vi "GCMBuilder.vi"() -> ()   [LabVIEW 2014]
uses:
  <vilib>/JKI/VIPM API/command-line/support/Version Info Cluster_vipm_api.ctl
  <vilib>/JKI/VIPM API/VIPM API_vipm_api.lvlib
panel:
  out "Build Output":path
  in  "Build":bool
  in  "VI Package Build Spec Data":T2
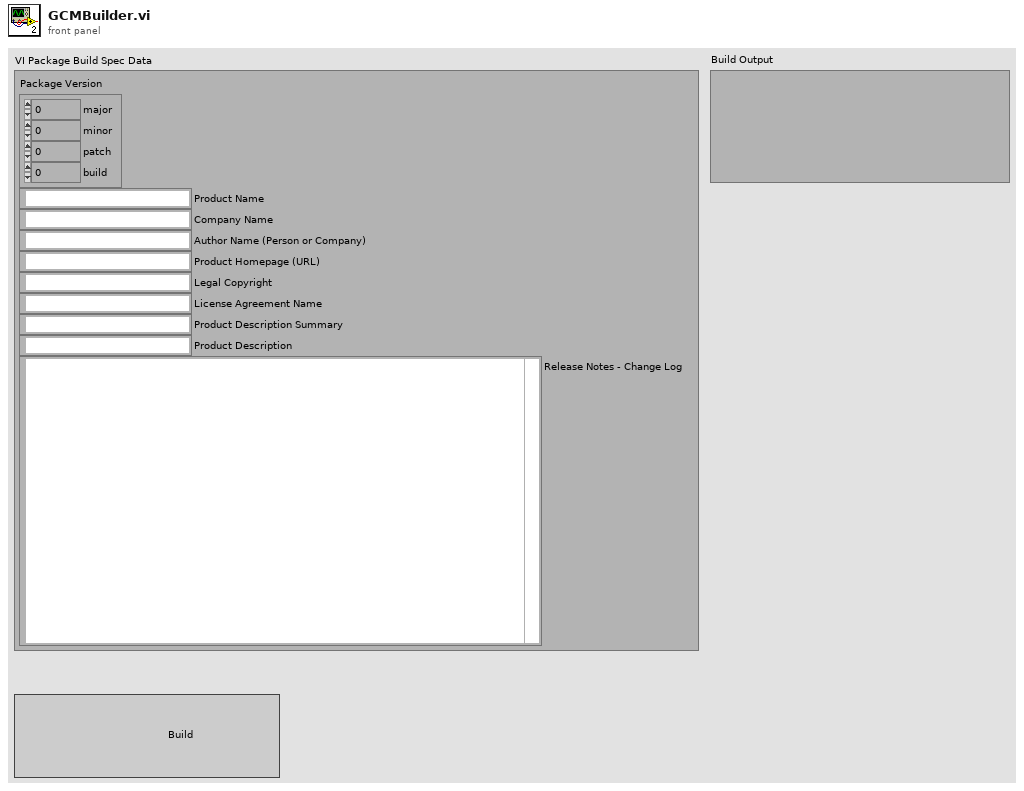
[diagram p1: front panel]
types:
  T1 = typedef "VIPM API_vipm_api.lvlib/Version Info Cluster_vipm_api.ctl" = cluster{"major":u32, "minor":u32, "patch":u32, "build":u32}
  T2 = cluster{"Package Version":T1, "Product Name":string, "Company Name":string, "Author Name (Person or Company)":string, "Product Homepage (URL)":string, "Legal Copyright":string, "License Agreement Name":string, "Product Description Summary":string, "Product Description":string, "Release Notes - Change Log":string}
  T3 = typedef "VIPM API_vipm_api.lvlib/VI Package Build Spec Data Cluster_vipm_api.ctl" = cluster{"Package Version":T1, "Product Name":string, "Company Name":string, "Author Name (Person or Company)":string, "Product Homepage (URL)":string, "Legal Copyright":string, "License Agreement Name":string, "Product Description Summary":string, "Product Description":string, "Release Notes - Change Log":string}
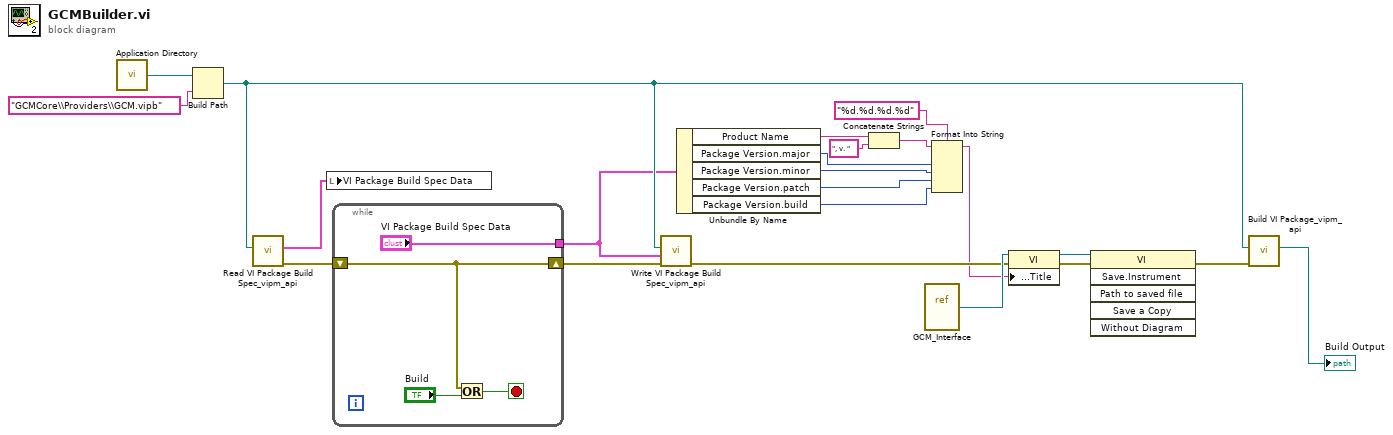
[diagram p0: block diagram]
diagram:
  n1 = call <vilib>:"Application Directory.vi"() -> ("Application Directory"=w22:path)
  n2 = Build Path(base path=w22, name or relative path="GCMCore\\Providers\\GCM.vipb") -> (appended path=w3:path)
  n3 = call <vilib>:"Read VI Package Build Spec_vipm_api.vi"("Path to VIPB File"=w3) -> ("error out"=w20:errorcluster, "VI Package Build Spec Data"=w4:T3)  [unwired: 9 in]
  n4 = local write "VI Package Build Spec Data"(w4) -> ()
  n5 = while {
    shift-right: [w26] -> w19
    shift-left: w20 -> [w26]
    tunnel: ["VI Package Build Spec Data"] -> w1
    stop <- w24 stop-if-true
    n6 = Or(x=w26, y="Build") -> (x .or. y?=w24:bool)
  }
  n7 = call <vilib>:"Write VI Package Build Spec_vipm_api.vi"("error in (no error)"=w19, "VI Package Build Spec Data"=w1, "Path to VIPB File"=w3) -> ("error out"=w10:errorcluster)  [unwired: 8 in]
  n8 = Unbundle By Name(w1) -> ("Product Name"=w16:string, "Package Version.major"=w11:u32, "Package Version.minor"=w12:u32, "Package Version.patch"=w13:u32, "Package Version.build"=w2:u32)
  n9 = Concatenate Strings(w16, ", v. ") -> (w15:string)
  n10 = vi-ref "GCM_Interface.vi"() -> (w18:refnum<vi>)
  n11 = Format Into String(format string="%d.%d.%d.%d", initial string=w15, w11, w12, w13, w2) -> (resulting string=w9:string)  [unwired: 1 in, 1 out]
  n12 = property class="VI"(reference=w18, error in=w10, "Front Panel.Title"=w9) -> (reference out=w8:refnum<vi>, error out=w7:errorcluster)
  n13 = invoke class="VI" method="Save.Instrument"(reference=w8, error in=w7) -> (error out=w6:errorcluster)  [unwired: 4 in, 5 out]
  n14 = call <vilib>:"Build VI Package_vipm_api.vi"("error in (no error)"=w6, "Path to VIPB File"=w3) -> ("Build Output"=→"Build Output":path)  [unwired: 8 in, 1 out]
